vi "Save_STS_ZSpecV2.vi"(9 "load":u16(ring) items=["Zspec_test"], 10 "stop":bool, 11 "Load":bool) -> (3 "Zspec Types []":string[](array[string]))   [LabVIEW 2014]
uses:
  <userlib>/Nanonis Prog Interface V5/Nanonis Prog Interface.lvlib
panel:
  out "data\n\n 2":T1(array[cluster])
  in  "ZspecParameters":T2 {"Threshold" min=-10 max=10 format="%#_6p"; "Sweep Distance (m)" min=-10 max=10 format="%#_6p"; "Initial Z-Offset (m)" min=-10 max=10 format="%#_6p"; "End of Sweep"."Z control time (s)" min=0 max=10 step=0.0001 format="%.3p"; "End of Sweep"."End settling time (s)" step=0.0001 format="%.3p"; "Sweep Timing"."Integration time (s)" min=0 max=20 step=0.0001 format="%.3p"; "Sweep Timing"."Settling time (s)" step=0.0001 format="%.3p"; "Sweep Timing"."Max. slew rate (V/s)" format="%.3p"; "Initialization"."Initial settling time (s)" step=0.0001 format="%.3p"; "Initialization"."Z averaging time (s)" min=0 max=10 step=0.0001 format="%.3p"; "Amplitude (mod. signal unit)" format="%#_6p"}
  out "loaded":i32
  in  "Save parameters":bool
  in  "Save As":string
  # "make sure\nLockin is activated\nin Advanced Settings"
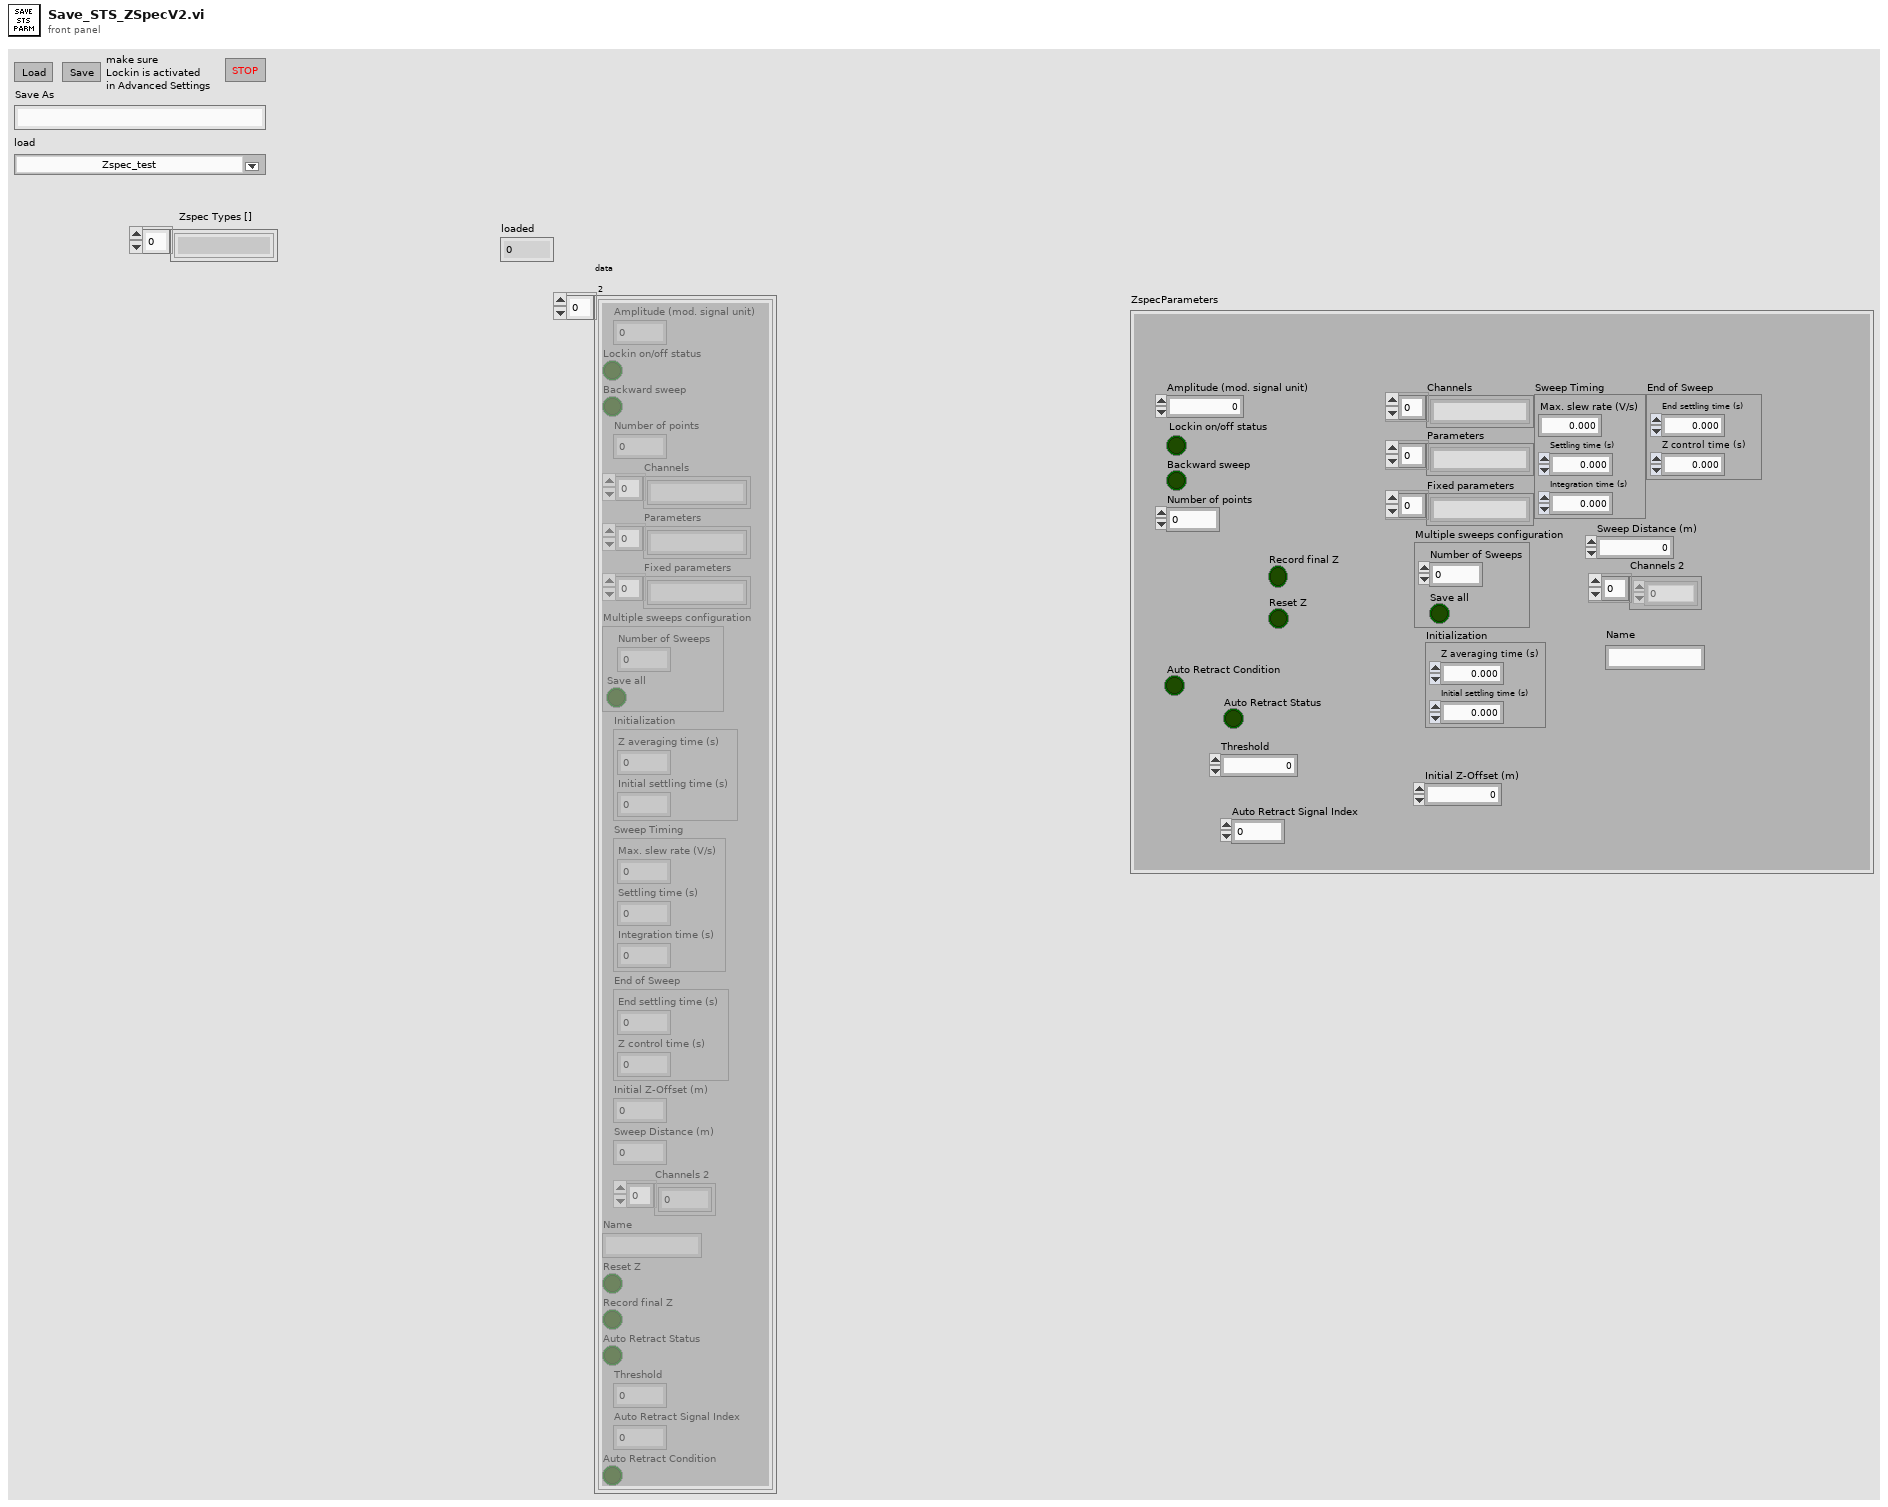
[diagram p1: front panel]
types:
  T1 = cluster{"Amplitude (mod. signal unit)":sgl, "Lockin on/off status":bool, "Backward sweep":bool, "Number of points":i32, "Channels":string[], "Parameters":string[], "Fixed parameters":string[], "Multiple sweeps configuration":cluster{"Number of Sweeps":i32, "Save all":bool}, "Initialization":cluster{"Z averaging time (s)":sgl, "Initial settling time (s)":sgl}, "Sweep Timing":cluster{"Max. slew rate (V/s)":sgl, "Settling time (s)":sgl, "Integration time (s)":sgl}, "End of Sweep":cluster{"End settling time (s)":sgl, "Z control time (s)":sgl}, "Initial Z-Offset (m)":sgl, "Sweep Distance (m)":sgl, "Channels 2":i32[], "Name":string, "Reset Z":bool, "Record final Z":bool, "Auto Retract Status":bool, "Threshold":sgl, "Auto Retract Signal Index":i32, "Auto Retract Condition":bool}[]
  T2 = cluster{"Amplitude (mod. signal unit)":sgl, "Lockin on/off status":bool, "Backward sweep":bool, "Number of points":i32, "Channels":string[], "Parameters":string[], "Fixed parameters":string[], "Multiple sweeps configuration":cluster{"Number of Sweeps":i32, "Save all":bool}, "Initialization":cluster{"Z averaging time (s)":sgl, "Initial settling time (s)":sgl}, "Sweep Timing":cluster{"Max. slew rate (V/s)":sgl, "Settling time (s)":sgl, "Integration time (s)":sgl}, "End of Sweep":cluster{"End settling time (s)":sgl, "Z control time (s)":sgl}, "Initial Z-Offset (m)":sgl, "Sweep Distance (m)":sgl, "Channels 2":i32[], "Name":string, "Reset Z":bool, "Record final Z":bool, "Auto Retract Status":bool, "Threshold":sgl, "Auto Retract Signal Index":i32, "Auto Retract Condition":bool}
  T3 = cluster{"Number of  Sweeps":i32, "Save all":bool}
  T4 = cluster{"Z averaging time (s)":sgl, "Initial settling time (s)":sgl}
  T5 = cluster{"Max. slew rate (m/s)":sgl, "Settling time (s)":sgl, "Integration time (s)":sgl}
  T6 = cluster{"End settling time (s)":sgl, "Z control time (s)":sgl}
  T7 = cluster{"Max. slew rate (V/s)":sgl, "Settling time (s)":sgl, "Integration time (s)":sgl}
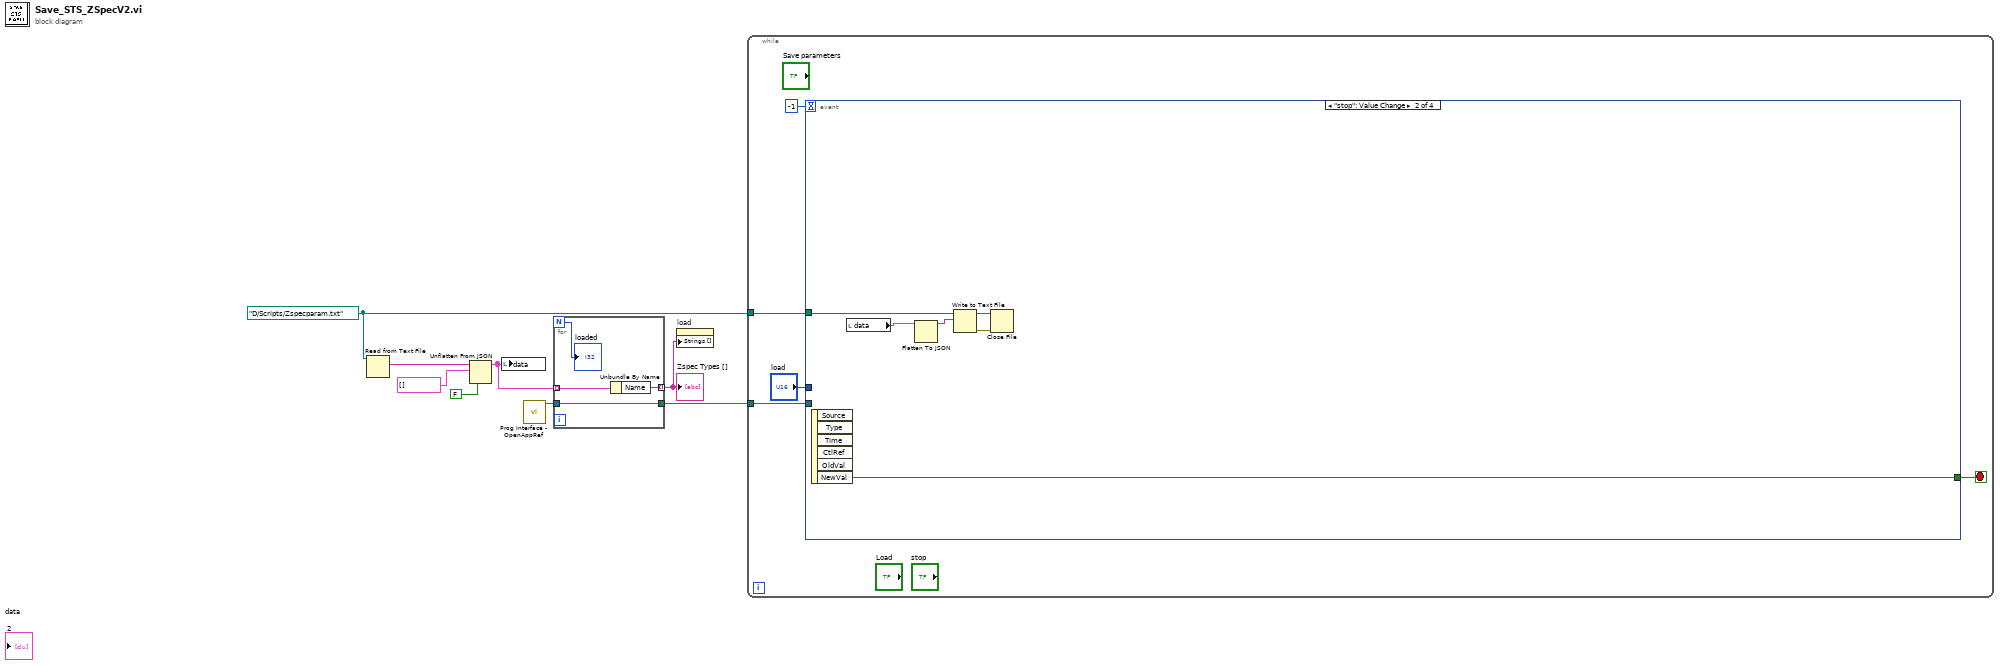
[diagram p0: block diagram]
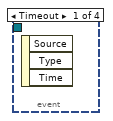
[diagram p2: hidden frame]
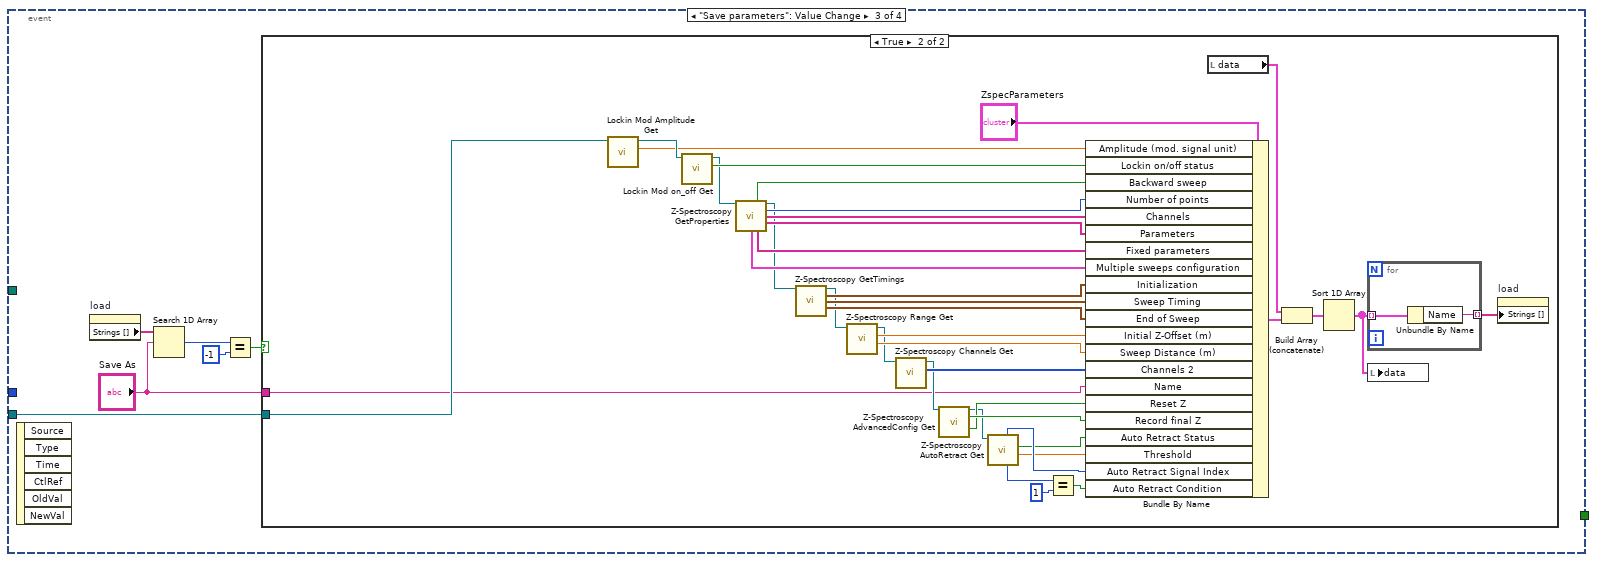
[diagram p3: hidden frame]
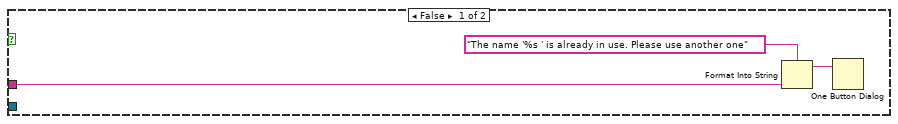
[diagram p4: hidden frame]
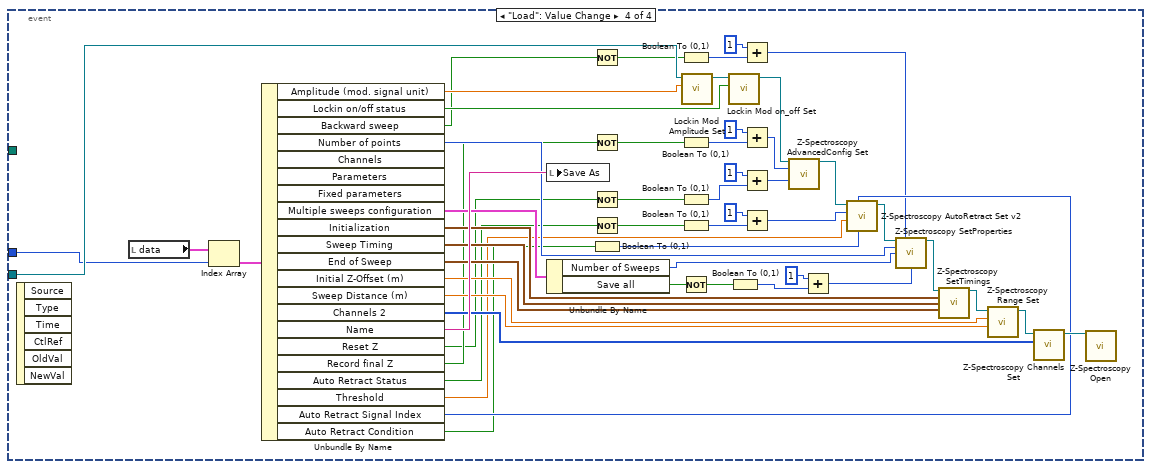
[diagram p5: hidden frame]
diagram:
  w8 = path "D:/Scripts/Zspecparam.txt" ("file (use dialog)")
  n1 = Read from Text File(file (use dialog)=w8) -> (text=w7:string)  [unwired: 3 in, 3 out]
  n2 = Unflatten From JSON(JSON string=w7, type and defaults=T1 [] ("data"), default null elements? (F)=FALSE) -> (value=w1:T1)  [unwired: 4 in, 1 out]
  n3 = local write "data\n\n 2"(w1) -> ()
  n4 = call <userlib>:"Prog Interface - OpenAppRef.vi"() -> ("Application reference"=w6:refnum<vi>)  [unwired: 6 in, 1 out]
  n5 = for {
    N -> [w9]
    tunnel: w1 -> [w12] mode=indexing
    tunnel: [w11] -> w3 mode=indexing
    tunnel: w6 -> [w10]
    tunnel: [w10] -> w5
    n6 = Unbundle By Name(w12) -> ("Name"=w11:string)
    "loaded" <- w9
  }
  "Zspec Types []" <- w3
  n7 = property on="load" class="Ring (strict)"("Strings []"=w3) -> ()  [unwired: 2 in, 2 out]
  n8 = while {
    tunnel: w5 -> [w17]
    tunnel: w8 -> [w14]
    stop <- w15 stop-if-true
    n9 = event shown="[1] \"stop\": Value Change" {
      selector: _ -> [_ _ _ _]
      dyn-events: _ -> [_ _ _ _]
      timeout: -1 -> [_ _ _ _]
      tunnel: w17 -> [_ _ w29 w123]
      tunnel: "load" -> [_ _ _ w118]
      tunnel: [_ w23 _ _] -> w15
      tunnel: w14 -> [_ w19 _ _]
      event Timeout {
        n10 = event-data() -> ()  [unwired: 1 in, 3 out]
      }
      event "stop": Value Change {
        n11 = event-data() -> ("NewVal"=w23:bool)  [unwired: 1 in, 5 out]
        n12 = local read "data\n\n 2"() -> (w18:T1)
        n13 = Flatten To JSON(anything=w18) -> (JSON string=w22:string)  [unwired: 2 in, 1 out]
        n14 = Write to Text File(file (use dialog)=w19, text=w22) -> (refnum out=w20:refnum<file>, error out=w21:errorcluster)  [unwired: 2 in, 1 out]
        n15 = Close File(refnum=w20, error in=w21) -> ()  [unwired: 2 out]
      }
      event "Save parameters": Value Change {
        n16 = event-data() -> ()  [unwired: 1 in, 6 out]
        n17 = property on="load" class="Ring (strict)"() -> ("Strings []"=w28:string[])  [unwired: 2 in, 2 out]
        n18 = Search 1D Array(1D array=w28, element="Save As") -> (index of element=w26:i32)  [unwired: 1 in]
        n19 = Equal?(x=w26, y=-1) -> (x = y?=w24:bool)
        n20 = case shown="True" w24 {
          tunnel: w29 -> [_ w69]
          tunnel: "Save As" -> [w32 w40]
          frame False {
            n21 = Format Into String(format string="The name '%s ' is already in use. Please use another one", w32) -> (resulting string=w30:string)  [unwired: 2 in, 1 out]
            n22 = One Button Dialog(message=w30) -> ()  [unwired: 1 in, 1 out]
          }
          frame True {
            n23 = call <userlib>:"Lockin Mod Amplitude Get.vi"("Application ref in"=w69) -> ("Amplitude (mod. signal unit)"=w65:sgl, "Application ref out"=w66:refnum<vi>)  [unwired: 8 in, 1 out]
            n24 = call <userlib>:"Lockin Mod on_off Get.vi"("Application ref in"=w66) -> ("Lockin on/off status"=w64:bool, "Application ref out"=w46:refnum<vi>)  [unwired: 8 in, 1 out]
            n25 = call <userlib>:"Z-Spectroscopy GetProperties.vi"("Application ref in"=w46) -> ("Backward sweep"=w63:bool, "Application ref out"=w45:refnum<vi>, "Number of points"=w62:i32, "Channels"=w61:string[], "Parameters"=w60:string[], "Multiple sweeps configuration"=w58:T3, "Fixed parameters"=w59:string[])  [unwired: 7 in, 1 out]
            n26 = call <userlib>:"Z-Spectroscopy GetTimings.vi"("Application ref in"=w45) -> ("Application ref out"=w44:refnum<vi>, "Initialization"=w57:T4, "Sweep Timing"=w56:T5, "End of Sweep"=w55:T6)  [unwired: 10 in, 1 out]
            n27 = call <userlib>:"Z-Spectroscopy Range Get.vi"("Application ref in"=w44) -> ("Z distance (m)"=w53:sgl, "Z offset (m)"=w54:sgl, "Application ref out"=w43:refnum<vi>)  [unwired: 6 in, 1 out]
            n28 = call <userlib>:"Z-Spectroscopy Channels Get.vi"("Application ref in"=w43) -> ("Channels"=w52:i8[], "Application ref out"=w42:refnum<vi>)  [unwired: 8 in, 1 out]
            n29 = call <userlib>:"Z-Spectroscopy AdvancedConfig Get.vi"("Application ref in"=w42) -> ("Application ref out"=w41:refnum<vi>, "Record final Z position at the end of the sweep"=w51:bool, "Reset Z at the end of the sweep"=w50:bool)  [unwired: 9 in, 3 out]
            n30 = call <userlib>:"Z-Spectroscopy AutoRetract Get.vi"("Application ref in"=w41) -> ("Threshold"=w47:sgl, "Auto retract status"=w48:bool, "Retract condition"=w35:enum16{">", "<"}, "Auto retract signal index"=w49:i32)  [unwired: 5 in, 2 out]
            n31 = Equal?(x=w35, y=1) -> (x = y?=w33:bool)
            n32 = Bundle By Name(cluster="ZspecParameters", "Amplitude (mod. signal unit)"=w65, "Lockin on/off status"=w64, "Backward sweep"=w63, "Number of points"=w62, "Channels"=w61, "Parameters"=w60, "Fixed parameters"=w59, "Multiple sweeps configuration"=w58, "Initialization"=w57, "Sweep Timing"=w56, "End of Sweep"=w55, "Initial Z-Offset (m)"=w54, "Sweep Distance (m)"=w53, "Channels 2"=w52, "Name"=w40, "Reset Z"=w50, "Record final Z"=w51, "Auto Retract Status"=w48, "Threshold"=w47, "Auto Retract Signal Index"=w49, "Auto Retract Condition"=w33) -> (w38:T2)
            n33 = local read "data\n\n 2"() -> (w37:T1)
            n34 = Build Array (concatenate)(w37, w38) -> (w68:T1)
            n35 = Sort 1D Array(array=w68) -> (sorted array=w36:T1)
            n36 = for {
              tunnel: w36 -> [w71] mode=indexing
              tunnel: [w70] -> w67 mode=indexing
              n37 = Unbundle By Name(w71) -> ("Name"=w70:string)
            }
            n38 = local write "data\n\n 2"(w36) -> ()
            n39 = property on="load" class="Ring (strict)"("Strings []"=w67) -> ()  [unwired: 2 in, 2 out]
          }
        }
      }
      event "Load": Value Change {
        n40 = event-data() -> ()  [unwired: 1 in, 6 out]
        n41 = local read "data\n\n 2"() -> (w124:T1)
        n42 = Index Array(array=w124, index=w118) -> (element=w102:T2)
        n43 = Unbundle By Name(w102) -> ("Amplitude (mod. signal unit)"=w115:sgl, "Lockin on/off status"=w116:bool, "Backward sweep"=w90:bool, "Number of points"=w103:i32, "Multiple sweeps configuration"=w109:cluster{"Number of Sweeps":i32, "Save all":bool}, "Initialization"=w112:T4, "Sweep Timing"=w113:T7, "End of Sweep"=w114:T6, "Initial Z-Offset (m)"=w106:sgl, "Sweep Distance (m)"=w107:sgl, "Channels 2"=w111:i32[], "Name"=w117:string, "Reset Z"=w76:bool, "Record final Z"=w79:bool, "Auto Retract Status"=w98:bool, "Threshold"=w94:sgl, "Auto Retract Signal Index"=w101:i32, "Auto Retract Condition"=w96:bool)  [unwired: 3 out]
        n44 = local write "Save As"(w117) -> ()
        n45 = Unbundle By Name(w109) -> ("Number of Sweeps"=w72:i32, "Save all"=w108:bool)
        n46 = Not(x=w90) -> (.not. x?=w91:bool)
        n47 = Not(x=w79) -> (.not. x?=w82:bool)
        n48 = Not(x=w76) -> (.not. x?=w77:bool)
        n49 = Not(x=w98) -> (.not. x?=w99:bool)
        n50 = Boolean To (0,1)(Boolean=w96) -> (0, 1=w95:i16)
        n51 = Boolean To (0,1)(Boolean=w91) -> (0, 1=w92:i16)
        n52 = Boolean To (0,1)(Boolean=w82) -> (0, 1=w83:i16)
        n53 = Boolean To (0,1)(Boolean=w77) -> (0, 1=w78:i16)
        n54 = Boolean To (0,1)(Boolean=w99) -> (0, 1=w100:i16)
        n55 = Not(x=w108) -> (.not. x?=w119:bool)
        n56 = call <userlib>:"Lockin Mod Amplitude Set.vi"("Amplitude (mod. signal unit)"=w115, "Application ref in"=w123) -> ("Application ref out"=w122:refnum<vi>)  [unwired: 8 in, 1 out]
        n57 = call <userlib>:"Lockin Mod on_off Set.vi"("Lockin ON/OFF"=w116, "Application ref in"=w122) -> ("Application ref out"=w84:refnum<vi>)  [unwired: 8 in, 1 out]
        n58 = Boolean To (0,1)(Boolean=w119) -> (0, 1=w121:i16)
        n59 = Add(x=i16 1, y=w92) -> (x+y=w88:i16)
        n60 = Add(x=i16 1, y=w83) -> (x+y=w81:i16)
        n61 = Add(x=i16 1, y=w78) -> (x+y=w74:i16)
        n62 = Add(x=i16 1, y=w100) -> (x+y=w97:i16)
        n63 = call <userlib>:"Z-Spectroscopy AdvancedConfig Set.vi"("Application ref in"=w84, "Record final Z position at the end of the sweep"=w81, "Reset Z at the end of the sweep"=w74) -> ("Application ref out"=w85:refnum<vi>)  [unwired: 11 in, 1 out]
        n64 = Add(x=i16 1, y=w121) -> (x+y=w73:i16)
        n65 = call <userlib>:"Z-Spectroscopy AutoRetract Set v2.vi"("Retract condition"=w95, "Auto retract signal index (-2=no change)"=w101, "Threshold"=w94, "Auto retract"=w97, "Application ref in"=w85) -> ("Application ref out"=w86:refnum<vi>)  [unwired: 5 in, 1 out]
        n66 = call <userlib>:"Z-Spectroscopy SetProperties.vi"("Application ref in"=w86, "Backward sweep"=w88, "Num points"=w103, "Num sweeps"=w72, "Save all sweeps (no change)"=w73) -> ("Application ref out"=w87:refnum<vi>)  [unwired: 9 in, 1 out]
        n67 = call <userlib>:"Z-Spectroscopy SetTimings.vi"("Application ref in"=w87, "Initialization (NaN)"=w112, "Sweep Timing (NaN)"=w113, "End of Sweep (NaN)"=w114) -> ("Application ref out"=w105:refnum<vi>)  [unwired: 10 in, 1 out]
        n68 = call <userlib>:"Z-Spectroscopy Range Set.vi"("Z distance (m)"=w107, "Z offset (m) (NaN=no change)"=w106, "Application ref in"=w105) -> ("Application ref out"=w104:refnum<vi>)  [unwired: 6 in, 1 out]
        n69 = call <userlib>:"Z-Spectroscopy Channels Set.vi"("Channels"=w111, "Application ref in"=w104) -> ("Application ref out"=w110:refnum<vi>)  [unwired: 8 in, 1 out]
        n70 = call <userlib>:"Z-Spectroscopy Open.vi"("Application ref in"=w110) -> ()  [unwired: 13 in, 2 out]
      }
    }
  }
